vi "get_by_timestamp.vi"(6 "tiebreak_right":i32=1, 8 "time_preference":i32, 9 "timestamp":u64, 10 "stream_handle":u64, 11 "path in":path=path "hl2ss_ulm.dll") -> (0 "packet":T1, 1 "packet_handle":u64, 2 "stream_handle":u64, 3 "path out":path)   [LabVIEW 2023]
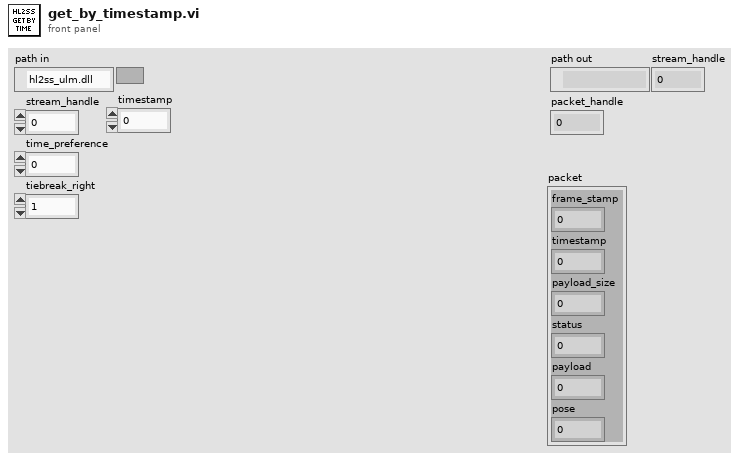
[diagram p1: front panel]
types:
  T1 = cluster{"frame_stamp":i64, "timestamp":u64, "payload_size":u32, "status":i32, "payload":u64, "pose":u64}
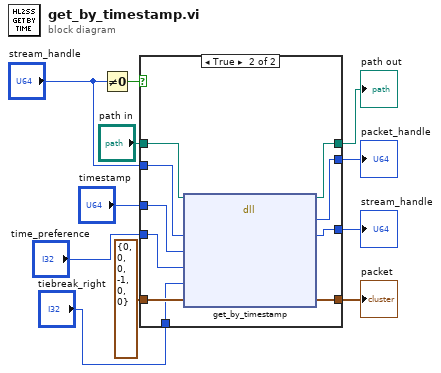
[diagram p0: block diagram]
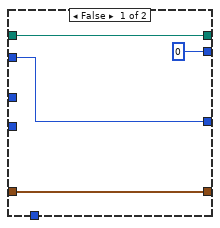
[diagram p2: hidden frame]
diagram:
  n1 = Not Equal To 0?(x="stream_handle") -> (x != 0?=w11:bool)
  n2 = case shown="True" w11 {
    tunnel: "path in" -> [w12 w25]
    tunnel: "stream_handle" -> [w14 w24]
    tunnel: "timestamp" -> [_ w23]
    tunnel: T1 {"frame_stamp"=0, "timestamp"=0, "payload_size"=0, "status"=-1, "payload"=0, "pose"=0} ("Cluster") -> [w15 w22]
    tunnel: [w12 w21] -> w7
    tunnel: [u64 0 ("return type") w20] -> w6
    tunnel: [w14 w19] -> w5
    tunnel: [w15 w18] -> w4
    tunnel: "time_preference" -> [_ w17]
    tunnel: "tiebreak_right" -> [_ w16]
    frame False {
    }
    frame True {
      n3 = dll-call lib="C:/Users/jcds/Documents/GitHub/hl2ss/extensions/client_labview/hl2ss_ulm.dll" fn="get_by_timestamp"(path in=w25, "handle"=w24, "timestamp"=w23, "time_preference"=w17, "tiebreak_right"=w16, "packet"=w22) -> (path out=w21:path, "return type"=w20:u64, "handle"=w19:u64, "packet"=w18:T1)  [unwired: 5 in, 1 out]
    }
  }
  "path out" <- w7
  "packet_handle" <- w6
  "stream_handle" <- w5
  "packet" <- w4
